vi "New.vi"(11 "TEMPLATE Msg Input in":refnum<class "TEMPLATE Msg Input.lvclass">) -> (0 "Error out":errorcluster, 3 "TEMPLATE Msg Input out":refnum<class "TEMPLATE Msg Input.lvclass">)   [LabVIEW 2020, in "_Template.lvlib" / "Templates.lvlib" / "TEMPLATE jettl Msg.lvlib" / "TEMPLATE Msg Input.lvclass"]
uses:
  TEMPLATE Msg Input.lvclass
  TEMPLATE Msg Input.lvclass/TEMPLATE Msg Input.ctl
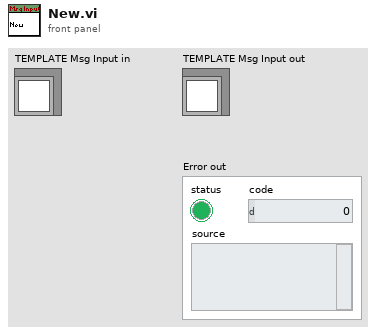
[diagram p1: front panel]
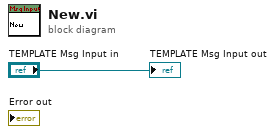
[diagram p0: block diagram]
diagram:
  "TEMPLATE Msg Input out" <- "TEMPLATE Msg Input in"
